vi "Write Previous Signal Configuration.vi"(8 "error in (no error)":errorcluster, 10 "previous signal configuration":refnum<class "SV Signal.lvclass">, 11 "current signal configuration in":refnum<class "SV Signal.lvclass">) -> (0 "error out":errorcluster, 3 "current signal configuration out":refnum<class "SV Signal.lvclass">)   [LabVIEW 2017, in "SV Signal.lvclass"]
uses:
  <vilib>/addons/_NISVFA/_Generation/Signal Generation/SV Signal/SV Signal.lvclass
  <vilib>/addons/_NISVFA/_Generation/Signal Generation/SV Signal/sv_Signal State Attribute.ctl
  <vilib>/addons/_NISVFA/_Generation/Signal Generation/SV Signal/SV Signal.lvclass/SV Signal.ctl
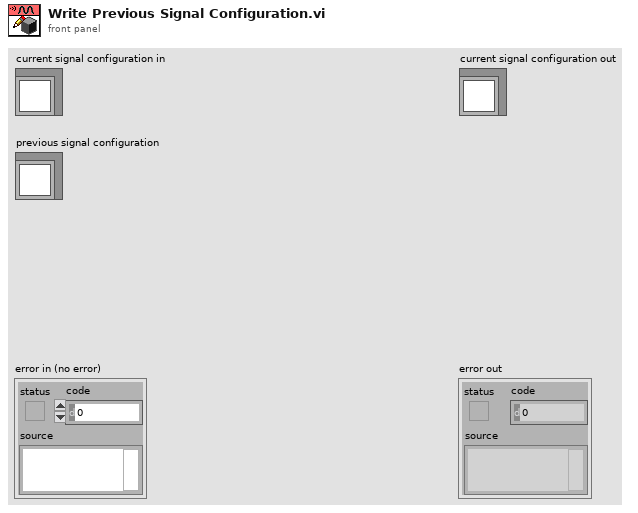
[diagram p1: front panel]
types:
  T1 = typedef "SV Signal.lvclass/sv_Signal State Attribute.ctl" = string
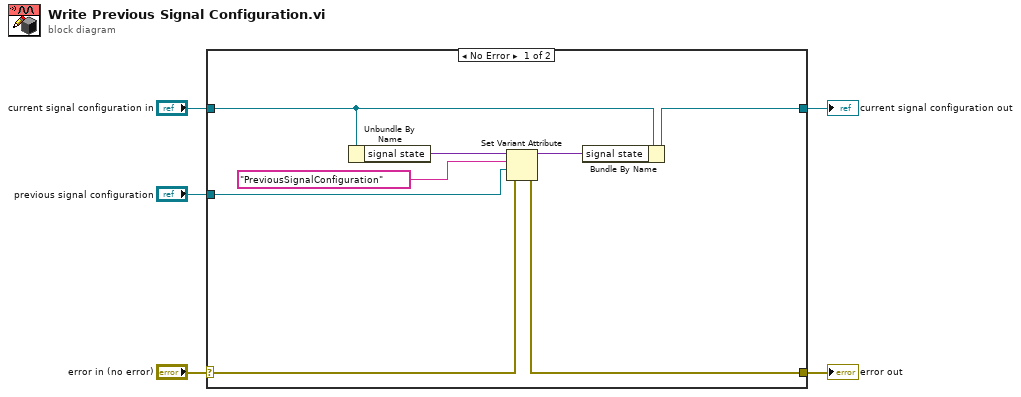
[diagram p0: block diagram]
diagram:
  n1 = case shown="No Error" "error in (no error)" {
    selector: "error in (no error)" -> [w11 w15]
    tunnel: [w10 w15] -> w4
    tunnel: [w6 w14] -> w2
    tunnel: "current signal configuration in" -> [w7 w14]
    tunnel: "previous signal configuration" -> [w9 _]
    frame No Error {
      n2 = Unbundle By Name(w7) -> ("signal state"=w13:variant)
      n3 = Set Variant Attribute(Variant=w13, name=T1 "PreviousSignalConfiguration", value=w9, error in=w11) -> (Variant out=w8:variant, error out=w10:errorcluster)  [unwired: 1 out]
      n4 = Bundle By Name(cluster=w7, "signal state"=w8) -> (w6:refnum<class "SV Signal.lvclass">)
    }
    frame Error {
    }
  }
  "error out" <- w4
  "current signal configuration out" <- w2
